vi "GLdrv_MEAS_OUTP_STAT.vi"(0 "Connection ID":T1, 11 "error in (no error)":errorcluster) -> (4 "Connection ID Out":T1, 6 "Buffer Size out":i32, 8 "Data No. out":i32, 10 "Break out":i32, 15 "error out":errorcluster)   [LabVIEW 2017, in "GL860_Driver.lvlib"]
doc: "リアルタイム転送の状況を参照します\nSTAT <BufferSize>,<DataNo>,<Break>\n<BufferSize>=バッファー内のデータ数\n<DataNo>=データナンバー\n<Break>=リアルタイムバッファから破棄されたデータ数"
uses:
  GL860_Driver.lvlib
  ConnectionID.ctl
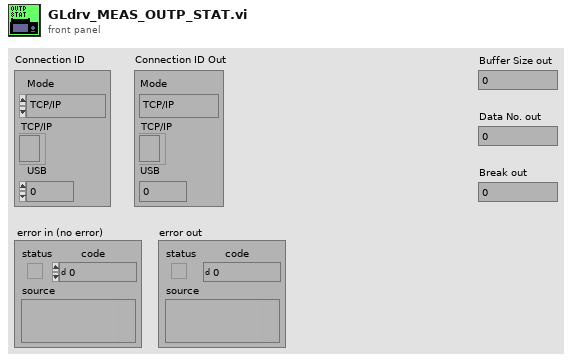
[diagram p1: front panel]
types:
  T1 = typedef "ConnectionID.ctl" = cluster{"Mode":enum16{"TCP/IP", "USB"}, "TCP/IP":refnum<k5>, "USB":i32}
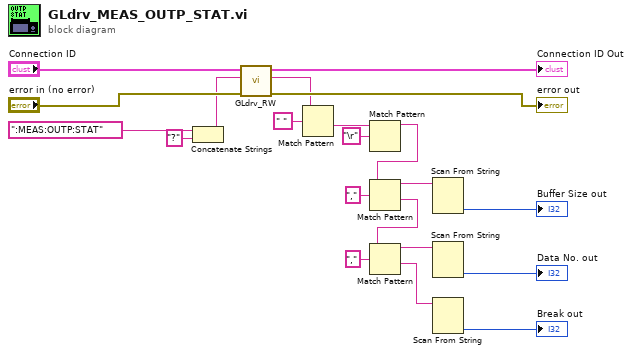
[diagram p0: block diagram]
diagram:
  n1 = Concatenate Strings(":MEAS:OUTP:STAT" ("Command"), "?" ("string")) -> (w11:string)
  n2 = call "GLdrv_RW.vi"("error in (no error)"="error in (no error)", "data in"=w11, "Connection ID"="Connection ID") -> ("error out"=→"error out":errorcluster, "data out"=w10:string, "Connection ID Out"=→"Connection ID Out":T1)  [unwired: 4 in, 2 out]
  n3 = Match Pattern(string=w10, regular expression=" " ("search string/char (-)")) -> (after substring=w13:string)  [unwired: 4 out]
  n4 = Match Pattern(string=w13, regular expression="\r") -> (before substring=w7:string)  [unwired: 4 out]
  n5 = Match Pattern(string=w7, regular expression=",") -> (before substring=w5:string, after substring=w6:string)  [unwired: 3 out]
  n6 = Match Pattern(string=w6, regular expression=",") -> (before substring=w4:string, after substring=w3:string)  [unwired: 3 out]
  n7 = Scan From String(input string=w5) -> (output 1=→"Buffer Size out":i32)  [unwired: 3 in, 4 out]
  n8 = Scan From String(input string=w4) -> (output 1=→"Data No. out":i32)  [unwired: 3 in, 4 out]
  n9 = Scan From String(input string=w3) -> (output 1=→"Break out":i32)  [unwired: 3 in, 4 out]
